vi "DAQNavi Read (Digital U8 1Chan 1Samp).vi"(8 "error in (no error)":errorcluster, 9 "portBit":i32=-1, 10 "timeout":dbl=10.0, 11 "task in":i32) -> (0 "error out":errorcluster, 2 "data":u8, 3 "task out":i32)   [LabVIEW 2020]
uses:
  DAQNavi_LV.dll
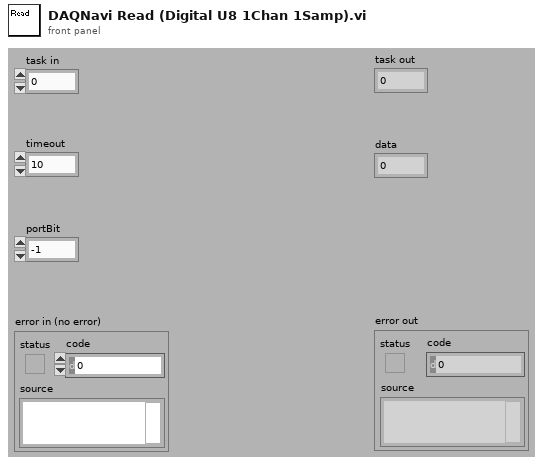
[diagram p1: front panel]
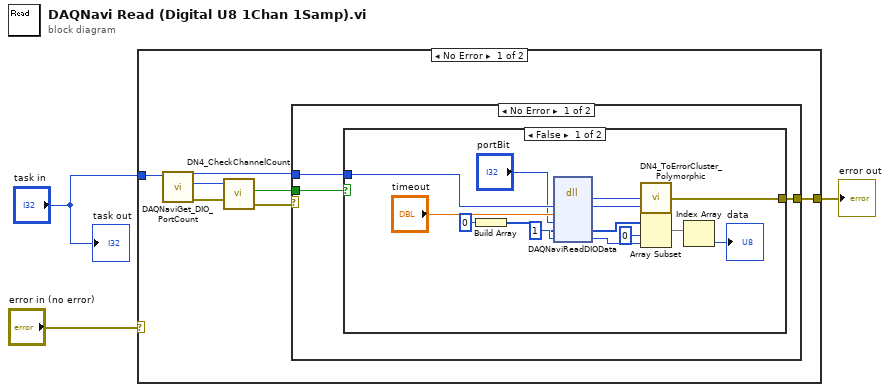
[diagram p0: block diagram]
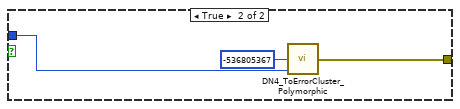
[diagram p2: hidden frame]
diagram:
  n1 = case shown="No Error" "error in (no error)" {
    selector: "error in (no error)" -> [_ w32]
    tunnel: "task in" -> [w10 _]
    tunnel: [w4 w32] -> w1
    frame No Error {
      n2 = call "DAQNaviGet_DIO_PortCount.vi"("task in"=w10) -> ("error out"=w9:errorcluster, "port count"=w8:i32, "task out"=w5:i32)  [unwired: 1 in, 7 out]
      n3 = call "DN4_CheckChannelCount.vi"("error out"=w9, "channel count"=w8) -> ("error IO"=w7:errorcluster, "greater than 1?"=w6:bool)  [unwired: 2 out]
      n4 = case shown="No Error" w7 {
        selector: w7 -> [_ w31]
        tunnel: [w13 w31] -> w4
        tunnel: w6 -> [w12 _]
        tunnel: w5 -> [w11 _]
        frame No Error {
          n5 = case shown="False" w12 {
            tunnel: [w25 w29] -> w13
            tunnel: w11 -> [w24 w28]
            frame False {
              n6 = Build Array(u8 0 ("element")) -> (w21:u8[])
              n7 = dll-call lib="DAQNavi_LV.dll" fn="DAQNaviReadDIOData"("taskID"=w24, "timeout"="timeout", "portBit"="portBit", "portData"=w21, "samples"=u32 1) -> ("return type"=w26:i32, "taskID"=w15:i32, "portData"=w20:u8[], "samples"=w18:u32)  [unwired: 5 in, 2 out]
              n8 = call "DN4_ToErrorCluster_Polymorphic.vi"("task id"=w15, "error code"=w26) -> ("error out"=w25:errorcluster)  [unwired: 3 out]
              n9 = Array Subset(array=w20, index=0, length=w18) -> (w17:u8[])
              n10 = Index Array(array=w17) -> (element=→"data":u8)  [unwired: 1 in]
            }
            frame True {
              n11 = call "DN4_ToErrorCluster_Polymorphic.vi"("task id"=w28, "error code"=-536805367 ("error code (0)")) -> ("error out"=w29:errorcluster)  [unwired: 3 out]
            }
          }
        }
        frame Error {
        }
      }
    }
    frame Error {
    }
  }
  "error out" <- w1
  "task out" <- "task in"
